vi "NI VeriStand - Specify Custom Device Execution Mode.vi"(7 "Execution Mode":T1, 8 "error in (no error)":errorcluster, 11 "Device Ref in":T2 format="%.0x") -> (0 "error out":errorcluster, 3 "Device Ref out":T2 format="%.0x")   [LabVIEW 2020, in "Custom Device API.lvlib"]
doc: "Specifies the execution mode of a custom device. Ensure the driver VI for the custom device is based on the template associated with the <B>Execution Mode</B> you specify."
uses:
  <vilib>/NI VeriStand/Custom Device API/Custom Device API.lvlib
  <vilib>/NI VeriStand/Custom Device API/Custom Device Item Ref.ctl
  <vilib>/NI VeriStand/Custom Device API/Custom Device Execution Mode.ctl
  073d8bc4-c213-4ba7-a3d1-4430157dfc8d.vi
  <vilib>/NI VeriStand/Custom Device API/Custom Device Offline Path.vi
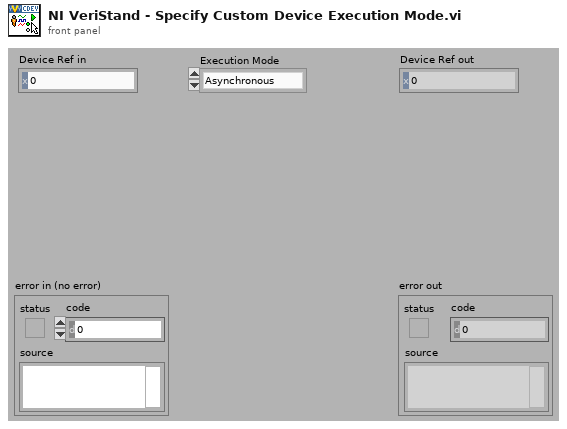
[diagram p1: front panel]
types:
  T1 = typedef "Custom Device API.lvlib/Custom Device Execution Mode.ctl" = enum16{"Asynchronous", "Inline HW Interface", "Inline Model Interface", "Inline Timing and Sync", "Asynchronous Timing and Sync"}
  T2 = typedef "Custom Device API.lvlib/Custom Device Item Ref.ctl" = u64
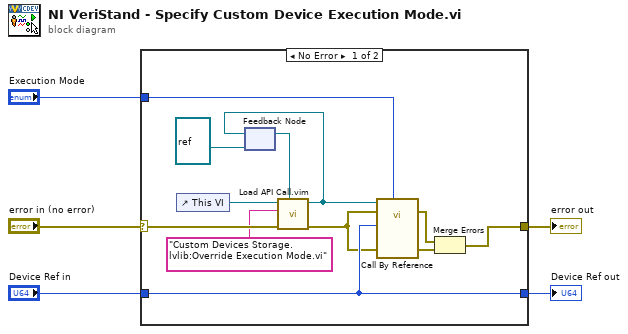
[diagram p0: block diagram]
diagram:
  n1 = case shown="No Error" "error in (no error)" {
    selector: "error in (no error)" -> [w11 w18]
    tunnel: [w16 w18] -> w5
    tunnel: "Execution Mode" -> [w15 _]
    tunnel: "Device Ref in" -> [w14 w19]
    tunnel: [w14 w19] -> w2
    frame No Error {
      n2 = control-ref of="This VI"() -> (w12:refnum<vi>)
      n3 = feedback #1(refnum<vi> refnum ("type specifier VI Refnum (for type only)")) -> (w13:refnum<vi>)
      n4 = call "Load API Call.vim"("VI reference in"=w13, "error in (no error)"=w11, "VI qualified name"="Custom Devices Storage.lvlib:Override Execution Mode.vi", "Caller VI ref"=w12) -> ("error out"=w10:errorcluster, "VI reference"=w9:refnum<vi>)  [unwired: 6 in]
      n5 = feedback-in #1(w9) -> ()
      n6 = call-by-ref "?"(reference=w9, error in=w10, "Execution Mode"=w15, 8:"error in (no error)"=w10, "Device Ref in"=w14) -> (error out=w6:errorcluster, 0:"error out"=w17:errorcluster)  [unwired: 7 in, 2 out]
      n7 = Merge Errors(w6, w17) -> (w16:errorcluster)
    }
    frame Error {
    }
  }
  "Device Ref out" <- w2
  "error out" <- w5
